vi "MICSD Do RSSI.vi"(7 "MICS Channel":u8, 8 "error in (no error)":errorcluster, 9 "Use Averaging?":bool=TRUE, 10 "RSSI Mode":u8, 11 "VISA Resource Name":refnum<visa-resource-name>) -> (0 "error out":errorcluster, 2 "RSSI VALUE":u16, 3 "dup VISA Resource Name":refnum<visa-resource-name>)   [LabVIEW 2010]
uses:
  <vilib>/Instr/_visa.llb/VISA Configure Serial Port (Instr).vi
panel:
  out "RAW RSSI Data":u16[](array[numeric])
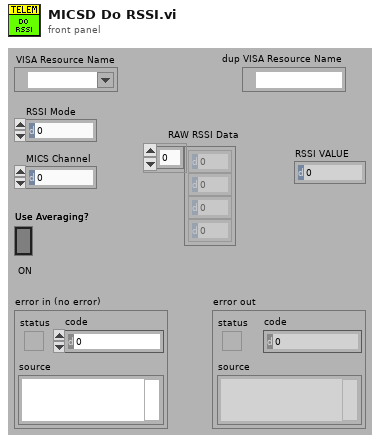
[diagram p1: front panel]
types:
  T1 = cluster{"Command Token":u8, "Length":u16, "Pack Data":u8[]}
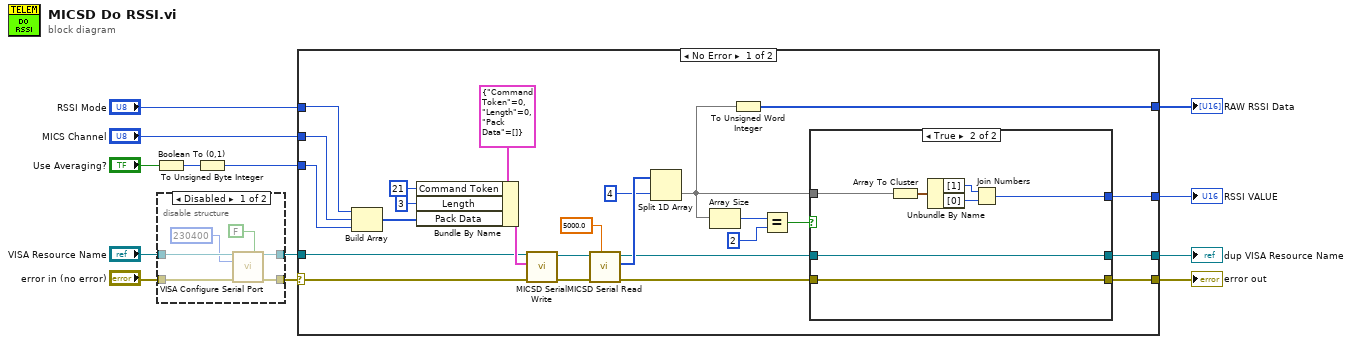
[diagram p0: block diagram]
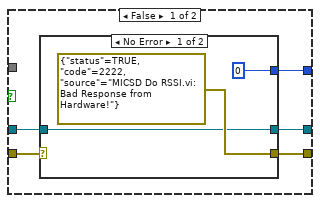
[diagram p3: hidden frame]
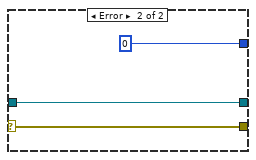
[diagram p4: hidden frame]
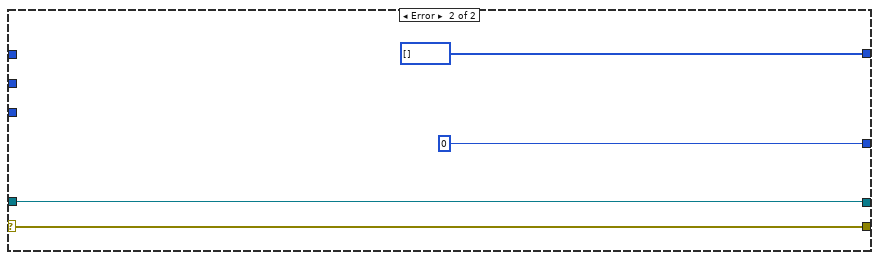
[diagram p5: hidden frame]
diagram:
  n1 = Boolean To (0,1)(Boolean="Use Averaging?") -> (0, 1=w5:i16)
  n2 = disable-structure shown="Disabled" {
    disable-tunnel: [w19 w20] -> w13
    disable-tunnel: [w18 w21] -> w12
    disable-tunnel: "VISA Resource Name" -> [w17 w21]
    disable-tunnel: "error in (no error)" -> [w16 w20]
    frame Disabled {
      n3 = call-poly "VISA Configure Serial Port"("VISA resource name"=w17, "Enable Termination\nChar (T)"=FALSE ("Enable Termination\nChar (T)"), "baud rate (9600)"=u32 230400, "error in (no error)"=w16) -> ("VISA resource name out"=w18:refnum<visa-resource-name>, "error out"=w19:errorcluster)  [unwired: 10 in]
    }
    frame Enabled {
    }
  }
  n4 = To Unsigned Byte Integer(number=w5) -> (unsigned 8bit integer=w4:u8)
  n5 = case shown="No Error" w13 {
    selector: w13 -> [w36 w68]
    tunnel: [w24 w68] -> w8
    tunnel: w12 -> [w37 w67]
    tunnel: [w26 w67] -> w9
    tunnel: [w31 u16[] []] -> w2
    tunnel: "RSSI Mode" -> [w34 _]
    tunnel: w4 -> [w33 _]
    tunnel: "MICS Channel" -> [w32 _]
    tunnel: [w29 u16 0] -> w1
    frame No Error {
      n6 = Build Array(w34, w32, w33) -> (w35:u8[])
      n7 = Bundle By Name(cluster=T1 {"Command Token"=0, "Length"=0, "Pack Data"=[]} ("Write Data"), "Command Token"=u8 21, "Length"=u16 3, "Pack Data"=w35) -> (w46:T1)
      n8 = call "MICSD Serial Write.vi"("error in (no error)"=w36, "Write Data"=w46, "VISA Resource Name"=w37) -> ("error out"=w41:errorcluster, "DUP Visa Resource Name"=w44:refnum<visa-resource-name>)  [unwired: 7 in]
      n9 = call "MICSD Serial Read.vi"("Timeout(mS)"=5000.0, "error in (no error)"=w41, "VISA Resource Name"=w44) -> ("error out"=w25:errorcluster, "Read Data"=w40:u8[], "DUP Visa Resource Name"=w27:refnum<visa-resource-name>)  [unwired: 6 in]
      n10 = Split 1D Array(array=w40, index=4) -> (second subarray=w30:u8[])  [unwired: 1 out]
      n11 = Array Size(array=w30) -> (size(s)=w23:i32)
      n12 = To Unsigned Word Integer(number=w30) -> (unsigned 16bit integer=w31:u16[])
      n13 = Equal?(x=w23, y=2) -> (x = y?=w28:bool)
      n14 = case shown="True" w28 {
        tunnel: w30 -> [_ w61]
        tunnel: [w51 w60] -> w29
        tunnel: w27 -> [w49 w59]
        tunnel: [w48 w59] -> w26
        tunnel: w25 -> [w47 w58]
        tunnel: [w50 w58] -> w24
        frame False {
          n15 = case shown="No Error" w47 {
            selector: w47 -> [_ w57]
            tunnel: [u16 0 u16 0] -> w51
            tunnel: [errorcluster {"status"=TRUE, "code"=2222, "source"="MICSD Do RSSI.vi: Bad Response from Hardware!"} ("error out") w57] -> w50
            tunnel: w49 -> [w52 w56]
            tunnel: [w52 w56] -> w48
            frame No Error {
            }
            frame Error {
            }
          }
        }
        frame True {
          n16 = Array To Cluster(array=w61) -> (cluster=w64:cluster{"[0]":u8, "[1]":u8})
          n17 = Unbundle By Name(w64) -> ("[1]"=w63:u8, "[0]"=w62:u8)
          n18 = Join Numbers(hi=w63, lo=w62) -> ((hi.lo)=w60:u16)
        }
      }
    }
    frame Error {
      (unwired) u16 0
    }
  }
  "dup VISA Resource Name" <- w9
  "error out" <- w8
  "RAW RSSI Data" <- w2
  "RSSI VALUE" <- w1
